vi "Initialize Path.vi"(8 "error in (no error)":errorcluster, 11 "Telegram Class in":refnum<class "Telegram Class.lvclass">) -> (0 "error out":errorcluster, 3 "Telegram Class out":refnum<class "Telegram Class.lvclass">)   [LabVIEW 2015, in "Telegram Library.lvlib" / "Telegram Class.lvclass"]
doc: "Created IvanLis by LabVIEW Portal\nProfile: http://labviewportal.org/memberlist.php?mode=viewprofile&u=987\neMail: IvanLisanov@gMail.com\nTelegram: https://t.me/IvanLis"
uses:
  Telegram Class.lvclass
  Telegram Class.lvclass/Telegram Class.ctl
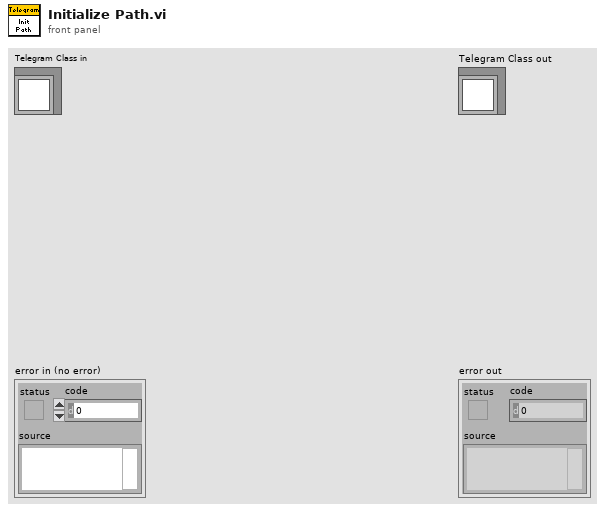
[diagram p1: front panel]
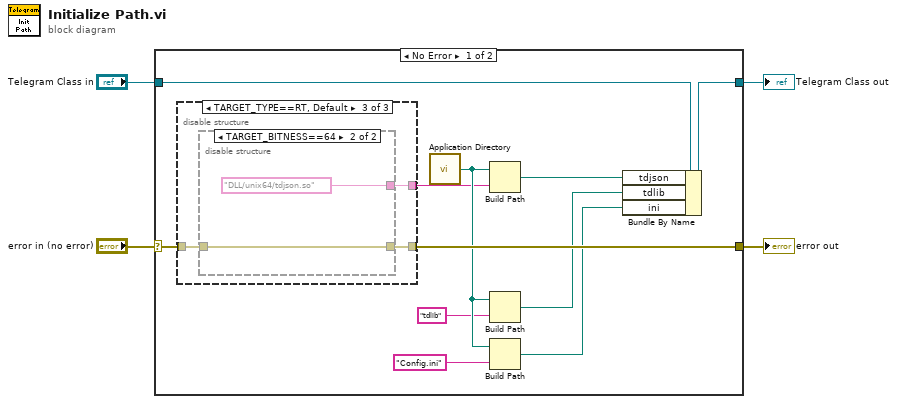
[diagram p0: block diagram]
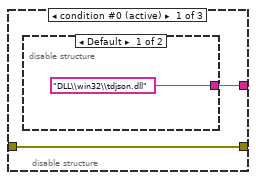
[diagram p2: hidden frame]
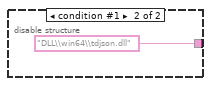
[diagram p3: hidden frame]
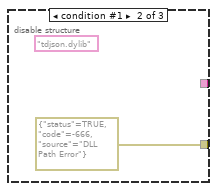
[diagram p4: hidden frame]
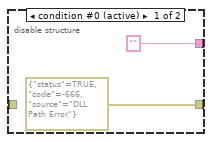
[diagram p5: hidden frame]
diagram:
  n1 = case shown="No Error" "error in (no error)" {
    selector: "error in (no error)" -> [w13 w29]
    tunnel: [w12 w29] -> w3
    tunnel: [w14 w28] -> w1
    tunnel: "Telegram Class in" -> [w15 w28]
    frame No Error {
      n2 = disable-structure shown="TARGET_TYPE==RT, Default" {
        disable-tunnel: w13 -> [w17 _ w23]
        disable-tunnel: [w17 errorcluster {"status"=TRUE, "code"=-666, "source"="DLL Path Error"} ("error IO") w22] -> w12
        disable-tunnel: [w16 _ w21] -> w7
        frame condition #0 (active) {
          n3 = disable-structure shown="Default" {
            disable-tunnel: ["DLL\\win32\\tdjson.dll" ("name or relative path") "DLL\\win64\\tdjson.dll" ("name or relative path")] -> w16
            frame condition #0 (active) {
            }
            frame condition #1 {
            }
          }
        }
        frame condition #1 {
          (unwired) "tdjson.dylib"
        }
        frame condition #2 {
          n4 = disable-structure shown="TARGET_BITNESS==64" {
            disable-tunnel: ["" ("name or relative path") "DLL/unix64/tdjson.so" ("name or relative path")] -> w21
            disable-tunnel: w23 -> [_ w26]
            disable-tunnel: [errorcluster {"status"=TRUE, "code"=-666, "source"="DLL Path Error"} ("error IO") w26] -> w22
            frame condition #0 (active) {
            }
            frame condition #1 {
            }
          }
        }
      }
      n5 = call <vilib>:"Application Directory.vi"() -> ("Application Directory"=w11:path)
      n6 = Build Path ("EXE include\nlocation")(base path=w11, name or relative path=w7) -> (appended path=w10:path)
      n7 = Build Path ("EXE include\nlocation")(base path=w11, name or relative path="tdlib") -> (appended path=w9:path)
      n8 = Build Path ("EXE include\nlocation")(base path=w11, name or relative path="Config.ini") -> (appended path=w8:path)
      n9 = Bundle By Name(cluster=w15, "tdjson"=w10, "tdlib"=w9, "ini"=w8) -> (w14:refnum<class "Telegram Class.lvclass">)
    }
    frame Error {
    }
  }
  "error out" <- w3
  "Telegram Class out" <- w1
